vi "EMV Draw Trigger Development Offline.vi"() -> ()   [LabVIEW 2016]
uses:
  type defs/EMV Flow Stop Detection.ctl
  Type Definitions/GEA3 HEWH ERD Data.ctl
  Type Definitions/GEA3 HEWH Mixing Valve.ctl
  <vilib>/Utility/file.llb/Read Delimited Spreadsheet (string).vi
panel:
  out "Algo Comparison":string[][](array[string])
  out "T6 Temp":string[](array[string])
  out "User Setpoint":string[](array[string])
  out "Flow State":string[](array[string])
  out "all rows":string[][](array[string])
  in  "file path (dialog if empty)":path=path "C:/Users/220038920/Desktop/Corey 2.csv"
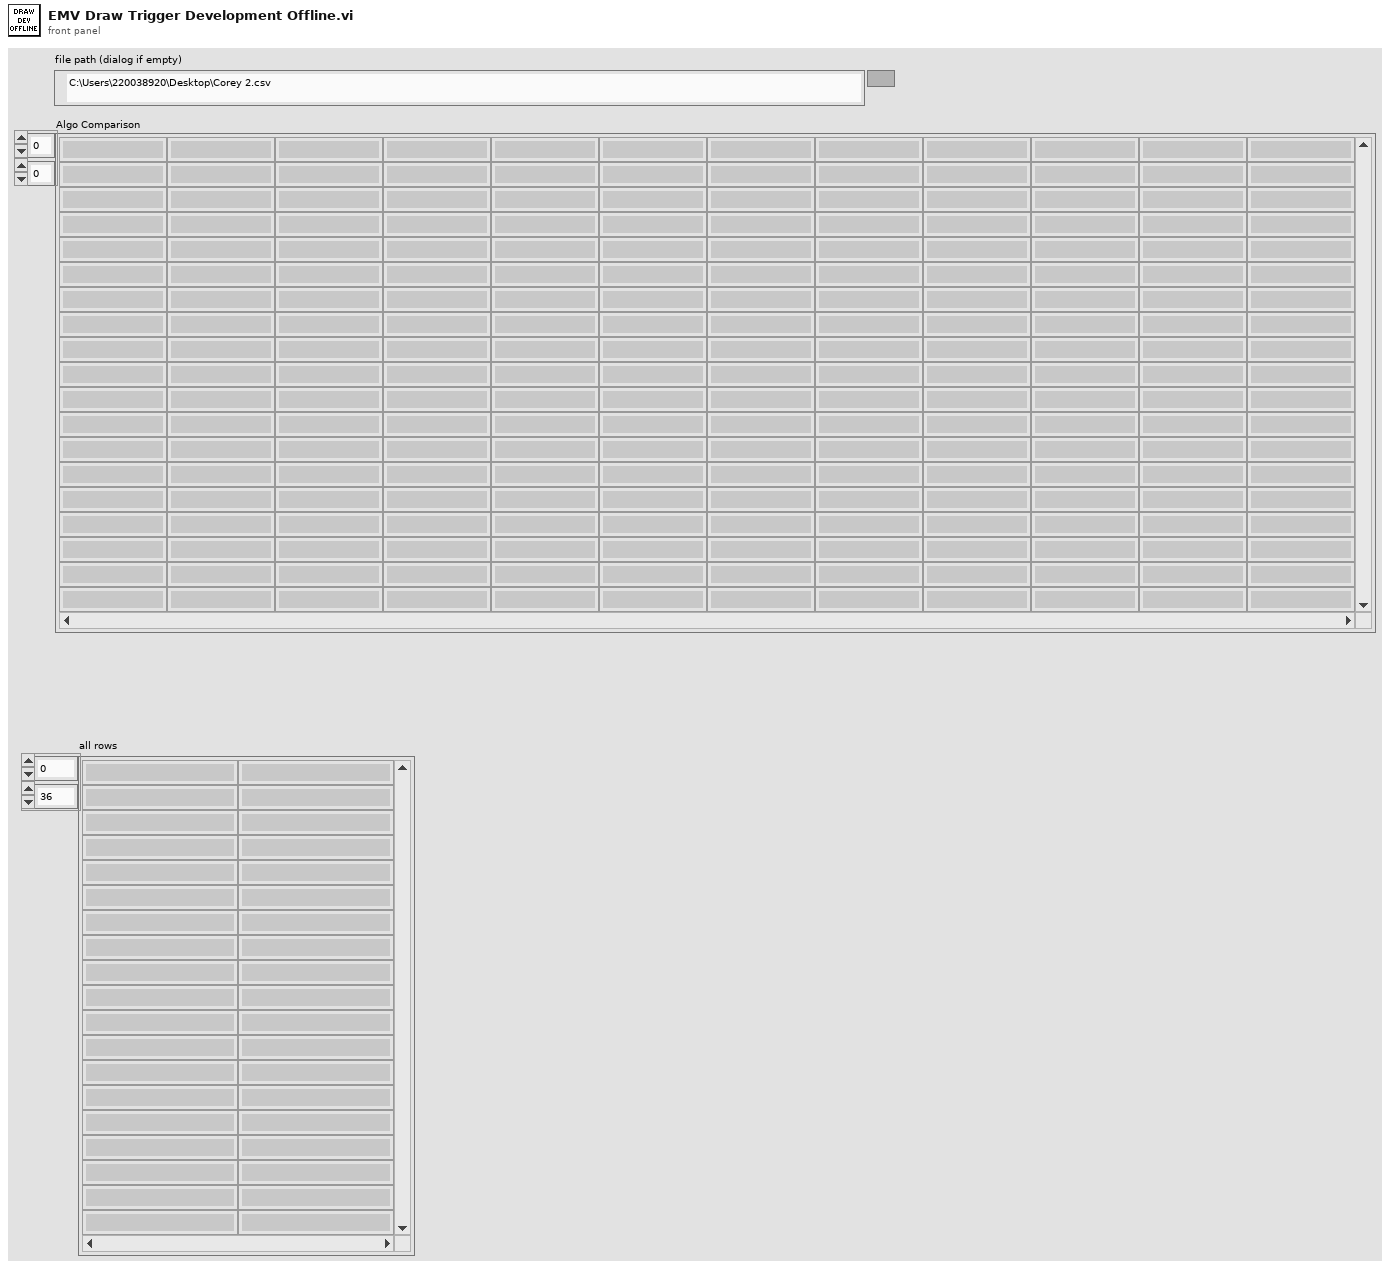
[diagram p1: front panel]
types:
  T1 = typedef "EMV Flow Stop Detection.ctl" = cluster{"UL Previous Position Slope":dbl, "UL Previous T6 Slope":dbl, "UL Previous Position":dbl, "UL Previous T6":dbl, "UL Current Position":dbl, "UL Current Position Slope":dbl, "UL Current T6":dbl, "UL Current T6 Slope":dbl, "New Algo End Of Flow":bool, "Start Up Timer":dbl, "Draw?":bool, "Disable F61":bool, "F61 Trip Old Algo":bool, "T6 + 8F":bool}
  T2 = typedef "GEA3 HEWH ERD Data.ctl" = cluster{"Mixing Valve":T3, "Standard ERDs":cluster{"User UI Mode (0X4020)":string, "User Setpoint (0x4024)":u16, "Actual Setpoint (0x4026)":u16, "DLB (0x4033)":bool, "Compressor (0x4033)":bool, "Lower Element (0x4033)":bool, "Upper Element (0x4033)":bool, "Fan (0x4033)":bool, "T1 Temp (0x405F)":dbl, "T2 Temp (0x4060)":dbl, "T3A Temp (0x4061)":dbl, "T3B Temp (0x4062)":dbl, "T4 Temp (0x4063)":dbl, "T5 Temp (0x4064)":dbl, "Line Voltage (0x4066)":dbl, "MeasuredCurrent (0x4065)":dbl, "LineVoltageTickCount(0x4007)":u16, "Number of Board Resets (0x412C)":u16, "T1 Temperature Raw (0x4016)":u16, "T2 Temperature Raw (0x4017)":u16}}
  T3 = typedef "GEA3 HEWH Mixing Valve.ctl" = cluster{"T7 Temp (0x40B9)":dbl, "MixValveStepOffset (0x400A)":i16, "MixValveAbsoluteStepPosition (0x400B)":i16, "Flow State (0x4009)":u8, "MixValveStepperControlOverride (0x400D)":string, "AverageInletSupplyTemperature (0x40B7)":dbl, "T6 Temp (0x406E)":dbl, "Kp Gain (0xF004)":u16, "Kp Qbits (0xF004)":u16, "Ki Gain (0xF004)":u16, "Ki Qbits (0xF004)":u16, "MixValveAbsoluteParkPosition(0x400C)":i16, "Day 2 Coldest T7 (0x40B1)":dbl, "Day 1 Coldest T7 (0x40B0)":dbl, "Day 4 Coldest T7 (0x40B3)":dbl, "Day 3 Coldest T7 (0x40B2)":dbl, "Day 6 Coldest T7 (0x40B5)":dbl, "Day 5 Coldest T7 (0x40B4)":dbl, "Average Inlet Supply T7 (0x40B7)":dbl, "Day 7 Coldest T7 (0x40B6)":dbl}
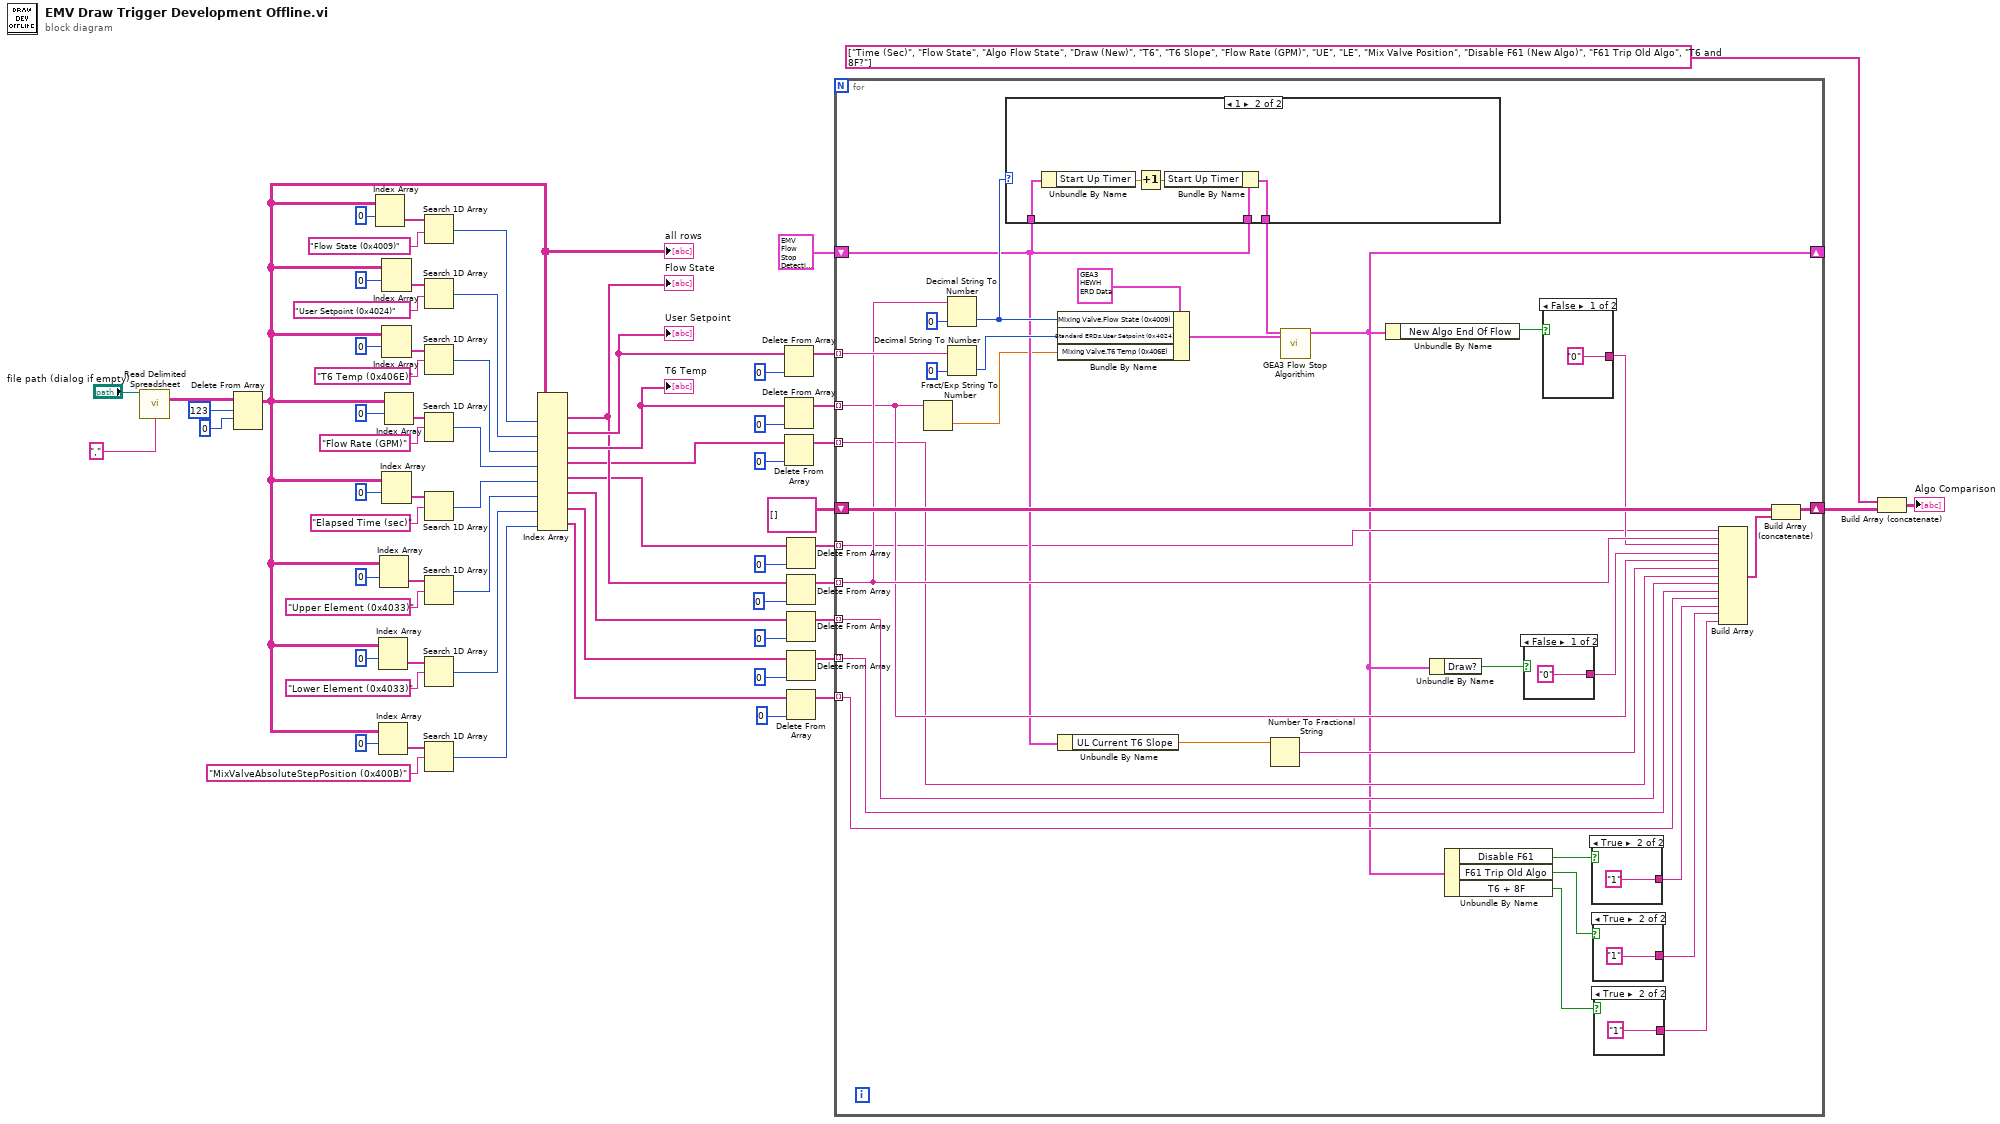
[diagram p0: block diagram]
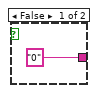
[diagram p2: hidden frame]
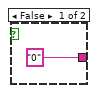
[diagram p3: hidden frame]
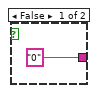
[diagram p4: hidden frame]
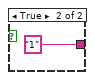
[diagram p5: hidden frame]
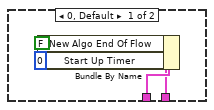
[diagram p6: hidden frame]
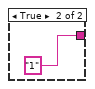
[diagram p7: hidden frame]
diagram:
  n1 = call-poly <vilib>:"Read Delimited Spreadsheet.vi"("file path (dialog if empty)"="file path (dialog if empty)", "delimiter (\\t)"="," ("delimiter (\\t)")) -> ("all rows"=w65:string[][])  [unwired: 8 in, 5 out]
  n2 = Delete From Array(array=w65, length=123, index (row)=0) -> (array with subset deleted=w3:string[][])  [unwired: 1 in, 1 out]
  "all rows" <- w3
  n3 = Index Array(array=w3, index (row)=0) -> (element=w33:string[])  [unwired: 1 in]
  n4 = Index Array(array=w3, index (row)=0) -> (element=w13:string[])  [unwired: 1 in]
  n5 = Index Array(array=w3, index (row)=0) -> (element=w9:string[])  [unwired: 1 in]
  n6 = Index Array(array=w3, index (row)=0) -> (element=w17:string[])  [unwired: 1 in]
  n7 = Index Array(array=w3, index (row)=0) -> (element=w29:string[])  [unwired: 1 in]
  n8 = Index Array(array=w3, index (row)=0) -> (element=w25:string[])  [unwired: 1 in]
  n9 = Index Array(array=w3, index (row)=0) -> (element=w21:string[])  [unwired: 1 in]
  n10 = Index Array(array=w3, index (row)=0) -> (element=w5:string[])  [unwired: 1 in]
  n11 = Search 1D Array(1D array=w33, element="Flow State (0x4009)") -> (index of element=w31:i32)  [unwired: 1 in]
  n12 = Search 1D Array(1D array=w29, element="User Setpoint (0x4024)") -> (index of element=w27:i32)  [unwired: 1 in]
  n13 = Search 1D Array(1D array=w25, element="T6 Temp (0x406E)") -> (index of element=w23:i32)  [unwired: 1 in]
  n14 = Search 1D Array(1D array=w5, element="Flow Rate (GPM)") -> (index of element=w2:i32)  [unwired: 1 in]
  n15 = Search 1D Array(1D array=w21, element="Elapsed Time (sec)") -> (index of element=w19:i32)  [unwired: 1 in]
  n16 = Search 1D Array(1D array=w17, element="Upper Element (0x4033)") -> (index of element=w15:i32)  [unwired: 1 in]
  n17 = Search 1D Array(1D array=w13, element="Lower Element (0x4033)") -> (index of element=w11:i32)  [unwired: 1 in]
  n18 = Search 1D Array(1D array=w9, element="MixValveAbsoluteStepPosition (0x400B)") -> (index of element=w7:i32)  [unwired: 1 in]
  n19 = Index Array(array=w3, index (col) #1=w31, index (col) #2=w27, index (col) #3=w23, index (col) #4=w2, index (col) #5=w19, index (col) #6=w15, index (col) #7=w11, index (col) #8=w7) -> (element #1=w50:string[], element #2=w58:string[], element #3=w59:string[], element #4=w47:string[], element #5=w1:string[], element #6=w41:string[], element #7=w40:string[], element #8=w36:string[])  [unwired: 8 in]
  "Flow State" <- w50
  "User Setpoint" <- w58
  "T6 Temp" <- w59
  n20 = Delete From Array(array=w58, index=0) -> (array with subset deleted=w57:string[])  [unwired: 1 in, 1 out]
  n21 = Delete From Array(array=w59, index=0) -> (array with subset deleted=w48:string[])  [unwired: 1 in, 1 out]
  n22 = Delete From Array(array=w47, index=0) -> (array with subset deleted=w46:string[])  [unwired: 1 in, 1 out]
  n23 = Delete From Array(array=w1, index=0) -> (array with subset deleted=w45:string[])  [unwired: 1 in, 1 out]
  n24 = Delete From Array(array=w50, index=0) -> (array with subset deleted=w51:string[])  [unwired: 1 in, 1 out]
  n25 = Delete From Array(array=w41, index=0) -> (array with subset deleted=w39:string[])  [unwired: 1 in, 1 out]
  n26 = Delete From Array(array=w40, index=0) -> (array with subset deleted=w38:string[])  [unwired: 1 in, 1 out]
  n27 = Delete From Array(array=w36, index=0) -> (array with subset deleted=w35:string[])  [unwired: 1 in, 1 out]
  n28 = for {
    tunnel: w51 -> [w92] mode=indexing
    tunnel: w57 -> [w99] mode=indexing
    tunnel: w48 -> [w84] mode=indexing
    shift-right: [w73] -> _
    shift-left: T1 {"UL Previous Position Slope"=0.0, "UL Previous T6 Slope"=0.0, "UL Previous Position"=0.0, "UL Previous T6"=0.0, "UL Current Position"=0.0, "UL Current Position Slope"=0.0, "UL Current T6"=0.0, "UL Current T6 Slope"=0.0, "New Algo End Of Flow"=FALSE, "Start Up Timer"=0.0, "Draw?"=FALSE, "Disable F61"=FALSE, "F61 Trip Old Algo"=FALSE, "T6 + 8F"=FALSE} ("Input") -> [w83]
    shift-right: [w93] -> w53
    shift-left: string[][] [] -> [w94]
    tunnel: w46 -> [w79] mode=indexing
    tunnel: w45 -> [w78] mode=indexing
    tunnel: w39 -> [w77] mode=indexing
    tunnel: w38 -> [w76] mode=indexing
    tunnel: w35 -> [w75] mode=indexing
    n29 = Fract/Exp String To Number(string=w84) -> (number=w80:dbl)  [unwired: 3 in, 1 out]
    n30 = Decimal String To Number(string=w92, default (0L)=u8 0 ("default (0 I32)")) -> (number=w87:u8)  [unwired: 1 in, 1 out]
    n31 = Decimal String To Number(string=w99, default (0L)=u16 0 ("default (0 I32)")) -> (number=w95:u16)  [unwired: 1 in, 1 out]
    n32 = case shown="1" w87 {
      tunnel: w83 -> [w112 w116]
      tunnel: [w111 w117] -> w89
      tunnel: w83 -> [_ w115]
      frame 0, Default {
        n33 = Bundle By Name(cluster=w112, "New Algo End Of Flow"=FALSE ("End Of Flow"), "Start Up Timer"=0) -> (w111:T1)
      }
      frame 1 {
        n34 = Unbundle By Name(w115) -> ("Start Up Timer"=w113:dbl)
        n35 = Increment(x=w113) -> (x+1=w114:dbl)
        n36 = Bundle By Name(cluster=w116, "Start Up Timer"=w114) -> (w117:T1)
      }
    }
    n37 = Bundle By Name(cluster=T2 {"Mixing Valve"={"T7 Temp (0x40B9)"=0.0, "MixValveStepOffset (0x400A)"=0, "MixValveAbsoluteStepPosition (0x400B)"=0, "Flow State (0x4009)"=0, "MixValveStepperControlOverride (0x400D)"="", "AverageInletSupplyTemperature (0x40B7)"=0.0, "T6 Temp (0x406E)"=0.0, "Kp Gain (0xF004)"=0, "Kp Qbits (0xF004)"=0, "Ki Gain (0xF004)"=0, "Ki Qbits (0xF004)"=0, "MixValveAbsoluteParkPosition(0x400C)"=0, "Day 2 Coldest T7 (0x40B1)"=0.0, "Day 1 Coldest T7 (0x40B0)"=0.0, "Day 4 Coldest T7 (0x40B3)"=0.0, "Day 3 Coldest T7 (0x40B2)"=0.0, "Day 6 Coldest T7 (0x40B5)"=0.0, "Day 5 Coldest T7 (0x40B4)"=0.0, "Average Inlet Supply T7 (0x40B7)"=0.0, "Day 7 Coldest T7 (0x40B6)"=0.0}, "Standard ERDs"={"User UI Mode (0X4020)"="", "User Setpoint (0x4024)"=0, "Actual Setpoint (0x4026)"=0, "DLB (0x4033)"=FALSE, "Compressor (0x4033)"=FALSE, "Lower Element (0x4033)"=FALSE, "Upper Element (0x4033)"=FALSE, "Fan (0x4033)"=FALSE, "T1 Temp (0x405F)"=0.0, "T2 Temp (0x4060)"=0.0, "T3A Temp (0x4061)"=0.0, "T3B Temp (0x4062)"=0.0, "T4 Temp (0x4063)"=0.0, "T5 Temp (0x4064)"=0.0, "Line Voltage (0x4066)"=0.0, "MeasuredCurrent (0x4065)"=0.0, "LineVoltageTickCount(0x4007)"=0, "Number of Board Resets (0x412C)"=0, "T1 Temperature Raw (0x4016)"=0, "T2 Temperature Raw (0x4017)"=0}} ("ERD Data"), "Mixing Valve.Flow State (0x4009)"=w87, "Standard ERDs.User Setpoint (0x4024)"=w95, "Mixing Valve.T6 Temp (0x406E)"=w80) -> (w96:T2)
    n38 = Unbundle By Name(w83) -> ("UL Current T6 Slope"=w82:dbl)
    n39 = Number To Fractional String(number=w82) -> (F-format string=w81:string)  [unwired: 3 in]
    n40 = call "GEA3 Flow Stop Algorithim.vi"("Input"=w89, "ERD Data"=w96) -> ("Output"=w73:T1)  [unwired: 16 in, 1 out]
    n41 = Unbundle By Name(w73) -> ("New Algo End Of Flow"=w88:bool)
    n42 = Unbundle By Name(w73) -> ("Draw?"=w86:bool)
    n43 = Unbundle By Name(w73) -> ("Disable F61"=w74:bool, "F61 Trip Old Algo"=w71:bool, "T6 + 8F"=w69:bool)
    n44 = case shown="False" w86 {
      tunnel: ["0" "1"] -> w85
      frame False {
      }
      frame True {
      }
    }
    n45 = case shown="False" w88 {
      tunnel: ["0" "1"] -> w91
      frame False {
      }
      frame True {
      }
    }
    n46 = case shown="True" w74 {
      tunnel: ["0" "1"] -> w72
      frame False {
      }
      frame True {
      }
    }
    n47 = case shown="True" w71 {
      tunnel: ["0" "1"] -> w70
      frame False {
      }
      frame True {
      }
    }
    n48 = case shown="True" w69 {
      tunnel: ["0" "1"] -> w68
      frame False {
      }
      frame True {
      }
    }
    n49 = Build Array(w78, w92, w91, w85, w84, w81, w79, w77, w76, w75, w72, w70, w68) -> (w90:string[])
    n50 = Build Array (concatenate)(w94, w90) -> (w93:string[][])
  }
  n51 = Build Array (concatenate)(string[] ["Time (Sec)", "Flow State", "Algo Flow State", "Draw (New)", "T6", "T6 Slope", "Flow Rate (GPM)", "UE", "LE", "Mix Valve Position", "Disable F61 (New Algo)", "F61 Trip Old Algo", "T6 and 8F?"], w53) -> (→"Algo Comparison":string[][])
